vi "TextFit_Insert Character Cluster array into Icon.vi"(4 "Max Width":i32, 5 "Color Set":T1={"BG"=65793, "FG"=239}, 6 "Starting Posiition":T6, 8 "Error":errorcluster, 10 "Character Array":T3[](array[typedef]), 11 "ICON":T2 caption="Icon") -> (0 "Error Out":errorcluster, 3 "ICON Out":T2)   [LabVIEW 2014]
doc: "Inserts the the Character Cluster array into the Icon at the given position"
uses:
  Controls/Cluster/Cluster_Top Left position.ctl
  Controls/Cluster/Cluster_Character Size and Priority Data.ctl
  Controls/String_Picture/String Char Normal.ctl
  Controls/Enum/ENUM_Font Size Select.ctl
  Controls/String_Picture/Picture_Icon.ctl
  Controls/Cluster/Cluster_Text Color Set.ctl
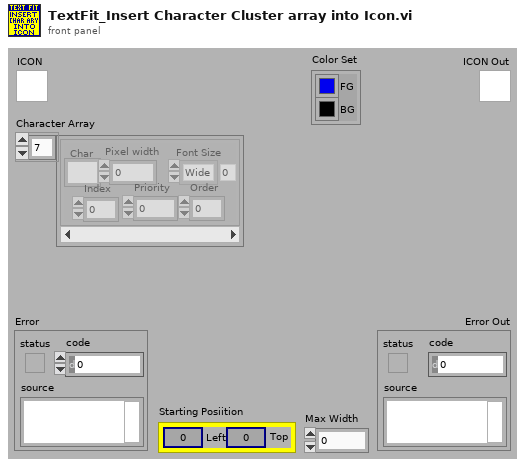
[diagram p1: front panel]
types:
  T1 = typedef "Cluster_Text Color Set.ctl" = cluster{"BG":u32, "FG":u32}
  T2 = typedef "Picture_Icon.ctl" = picture
  T3 = typedef "Cluster_Character Size and Priority Data.ctl" = cluster{"Char":T4, "Font Size":T5, "Pixel width":i32, "Priority":i32, "Order":i32, "Index":i32}
  T4 = typedef "String Char Normal.ctl" = string
  T5 = typedef "ENUM_Font Size Select.ctl" = enum16{"Wide", "Med", "Thin"}
  T6 = typedef "Cluster_Top Left position.ctl" = cluster{"Left":i32, "Top":i32}
  T7 = typedef "Array Bool Char Bits Wide.ctl" = bool[][]
  T8 = typedef "imagedata.ctl" = cluster{"image type":i32, "image depth":i32, "image":u8[], "mask":u8[], "colors":u32[], "Rectangle":cluster{"left":i16, "top":i16, "right":i16, "bottom":i16}}
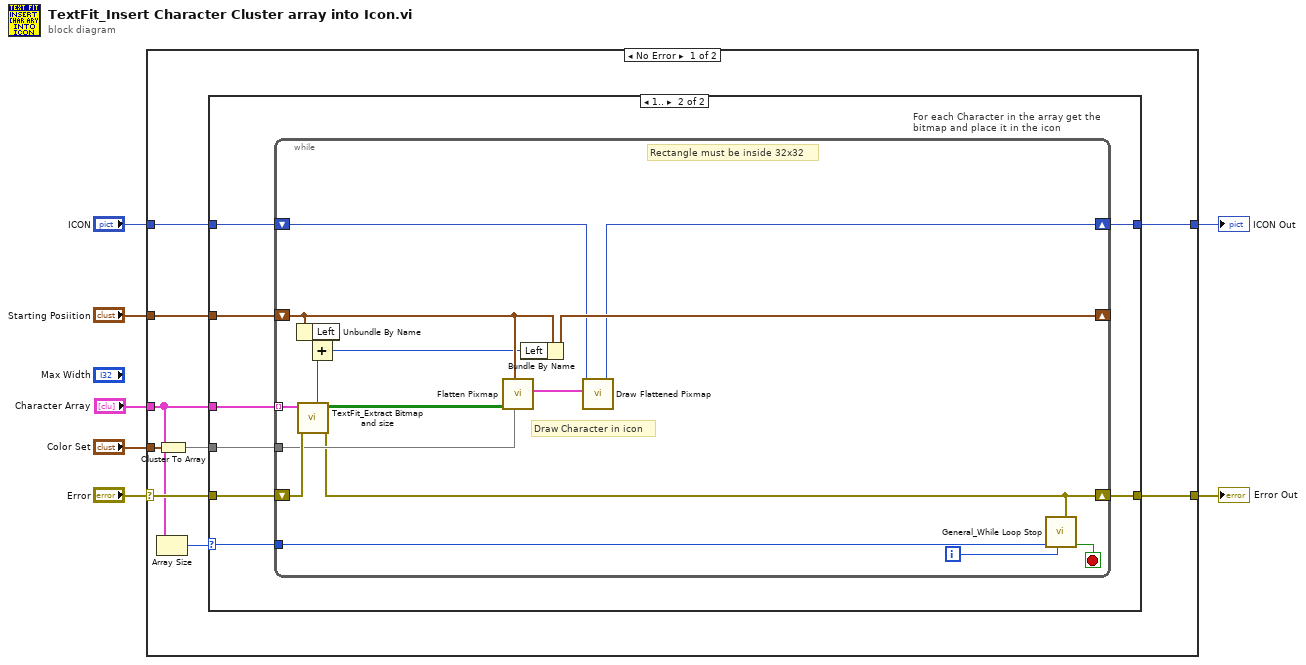
[diagram p0: block diagram]
diagram:
  n1 = case shown="No Error" "Error" {
    selector: "Error" -> [w11 w43]
    tunnel: [w16 w43] -> w7
    tunnel: "Starting Posiition" -> [w9 _]
    tunnel: "Character Array" -> [w10 _]
    tunnel: [w15 w44] -> w4
    tunnel: "ICON" -> [w14 w44]
    tunnel: "Color Set" -> [w13 _]
    frame No Error {
      n2 = Array Size(array=w10) -> (size(s)=w8:i32)
      n3 = Cluster To Array(cluster=w13) -> (array=w12:u32[])
      n4 = case shown="1.." w8 {
        selector: w8 -> [_ w19]
        tunnel: [w18 w26] -> w16
        tunnel: [w17 w25] -> w15
        tunnel: w14 -> [w17 w24]
        tunnel: w12 -> [_ w23]
        tunnel: w11 -> [w18 w22]
        tunnel: w10 -> [_ w21]
        tunnel: w9 -> [_ w20]
        frame ..0 {
        }
        frame 1.. {
          n5 = while "For each Character in the array get the \nbitmap and place it in the icon" {
            shift-right: [w38] -> w25
            shift-left: w24 -> [w37]
            shift-right: [w42] -> _
            shift-left: w20 -> [w36]
            tunnel: w21 -> [w40] mode=indexing
            shift-right: [w33] -> w26
            shift-left: w22 -> [w41]
            tunnel: w23 -> [w34]
            tunnel: w19 -> [w28]
            i -> [w29]
            stop <- w30 stop-if-true
            # "Draw Character in icon"
            # "Rectangle must be inside 32x32"
            n6 = Unbundle By Name(w36) -> ("Left"=w32:i32)
            n7 = call "TextFit_Extract Bitmap and size.vi"("Error"=w41, "Character Cluster"=w40) -> ("Error Out"=w33:errorcluster, "BitMap Out"=w35:T7, "Size Out"=w39:i32)  [unwired: 7 in]
            n8 = Add(x=w32, y=w39) -> (x+y=w31:i32)
            n9 = call <vilib>:"Flatten Pixmap.vi"("colors"=w34, "top left"=w36, "1-bit pixmap"=w35) -> ("image data"=w27:T8)  [unwired: 8 in]
            n10 = Bundle By Name(cluster=w36, "Left"=w31) -> (w42:T6)
            n11 = call <vilib>:"Draw Flattened Pixmap.vi"("image data"=w27, "picture"=w37) -> ("new picture"=w38:picture)  [unwired: 7 in]
            n12 = call "General_While Loop Stop.vi"("Error In"=w33, "Index In"=w29, "Array Size In"=w28) -> ("Stop Out3"=w30:bool)  [unwired: 4 in, 3 out]
          }
        }
      }
    }
    frame Error {
    }
  }
  "Error Out" <- w7
  "ICON Out" <- w4
